vi "Calculate_WDID.vi"() -> ()   [LabVIEW 2012]
panel:
  in  "SID":u32=9
  in  "ST":u32=12
  in  "DT":u32
  in  "DU":u32=17
  in  "CV":u32
  out "WDID (binair)":u32 format="%032b"
  out "WDID (decimal)":u32
  # "This VI calculates WDID-word (32 bits unsigned integer)."
  # "// Creates a Weather Data ID from the components\n#define MAKE_WDID(CV, DU, DT, ST, SID)  ( ((CV) & 0x1F) | (((DU) & 0x1F)<<5) | (((DT) & 0x1F)<<10) | (((ST) & 0xFF)<<16) | (((SID) & 0xFF) <<24) )\n\n// Weather Data ID field values\n\n// Calculated Variable - 5 bits        // Input parameters\n#define WDAT_CV_DIRECT_DATA      (0)   // NOT a calculated value, \n                                       // 0=SID   1=ST\n#define WDAT_CV_DEWPOINT         (1)   // 0-Temp, 1-Humidity\n#define WDAT_CV_WINDCHILL        (2)   // 0-Temp,             Implied: Wind Speed\n#define WDAT_CV_HEAT             (3)   // 0-Temp, 1-Humidity\n#define WDAT_CV_THWINDEX         (4)   // 0-Temp, 1-Humidity, Implied: Wind Speed\n#define WDAT_CV_THSWINDEX        (5)   // 0-Temp, 1-Humidity, Implied: Speed, Solar, Time/Location\n#define WDAT_CV_WETBULB          (6)   // 0-Temp, 1-Humidity\n#define WDAT_CV_WINDRUN          (7)   //                     Implied: Speed, Arc Interval\n#define WDAT_CV_DEGDAYS_INTEG    (8)   // 0-Temp, 1-Threshold Implied: Arc Interval\n#define WDAT_CV_SOLAR_ENERGY     (9)   //                     Implied: Solar, Arc Interval\n#define WDAT_CV_UV_DOSE          (10)  //                     Implied: UV, Arc Interval\n#define WDAT_CV_AIR_DENSITY      (11)  // 0-Temp, 1-Humidity  Implied barometer\n#define WDAT_CV_EMC              (12)  // 0-Temp, 1-Humidity\n#define WDAT_CV_ET               (13)  // This is calculated on the Vantage, but does not have \n                                       // a particular sensor to file it under\n#define WDAT_CV_DEGDAYS_HI_LOW   (14)  // 0-Temp, 1-Threshold Implied: Arc Interval\n\n// Display Units - 5 bits - This is NOT an independant variable\n#define WDAT_DU_TEMP_DEG         (0)   // Degrees of Temperature (F,C)\n#define WDAT_DU_DEG_DAYS         (1)   // Degrees of Temp Accumulation (0F = 0C)\n#define WD0      (2)   // Water Accumulation (Rain, ET) (in,mm)\n#define WDAT_DU_WATER_ACCUM      (2)   // Water Accumulation (Rain, ET) (in,mm) -- another define\n#define WDAT_DU_WATER_RATE       (3)   // Water Rate (in/hr, mm/hr)\n#define WDAT_DU_SPEED            (4)   // Wind Speed (mph,kt,kph,m/s)\n#define WDAT_DU_DIR_DEG          (5)   // Wind Direction in degrees \n#define WDAT_DU_DIR_SECTOR       (6)   // Wind Direction in sector code\n#define WDAT_DU_PRESSURE         (7)   // Air Pressure (in Hg, mm Hg, mb)\n#define WDAT_DU_TIME             (8)   // Time of Day (12hr, 24hr)\n#define WDAT_DU_TIME_ACCUM       (9)   // Accumulated # minutes\n#define WDAT_DU_SOLAR_RAD        (10)  // Solar Rad (W/m^2)\n#define WDAT_DU_SOLAR_ENERGY     (11)  // Solar Energy (Ly)\n#define WDAT_DU_UV_INDEX         (12)  // UV radiation (Index)\n#define WDAT_DU_UV_DOSE          (13)  // UV Dose (MEDs)\n#define WDAT_DU_PERCENT          (14)  // Percentage (i.e. Relative Hum) (%)\n#define WDAT_DU_SOIL_MOISTURE    (15)  // Wetness of the Soil (cb)\n#define WDAT_DU_LEAF_WET         (16)  // Wetness of Leaf surface (0-15)\n#define WDAT_DU_SCALAR           (17)  // Dimensionless numbers (Reed Open, nSamples, etc)\n#define WDAT_DU_DISTANCE         (18)  // Miles, Km, etc for Wind run\n#define WDAT_DU_ELEVATION        (19)  // Feet or Meters. for Bar Calibration etc\n#define WDAT_DU_AIR_DENSITY      (20)  // Air density units\n#define WDAT_DU_BAR_TREND        (21)  // barometer trend (5-position)\n\n// Data Type - 5 bits\n#define WDAT_DT_CURRENT          (0)   // Current instantanious value\n//#define WDAT_DT_ARC_ACCUM        (1)   // Accumulation over the archive interval\n//#define WDAT_DT_HIGH             (2)   // High within an archive interval\n//#define WDAT_DT_LOW              (3)   // Low within an archive interval\n#define WDAT_DT_DAY_HIGH         (4)   // Daily High\n//#define WDAT_DT_DAY_HIGH_TIME    (5)   // Time of Daily High\n#define WDAT_DT_DAY_LOW          (6)   // Daily Low\n//#define WDAT_DT_DAY_LOW_TIME     (7)   // Time of Daily Low\n#define WDAT_DT_DAY_AVERAGE      (8)   // Daily Average\n#define WDAT_DT_DAY_ACCUM        (9)   // Daily Accumulation\n#define WDAT_DT_MONTH_HIGH       (10)  // Monthly High\n//#define WDAT_DT_MONTH_HIGH_TIME  (11)  // Time of Monthly High\n#define WDAT_DT_MONTH_LOW        (12)  // Monthly Low\n//#define WDAT_DT_MONTH_LOW_TIME   (13)  // Time of Monthly Low\n//#define WDAT_DT_MONTH_AVERAGE    (14)  // Monthly Average\n//#define WDAT_DT_MONTH_AVG_HIGH   (15)  // Monthly Average of Daily Highs\n//#define WDAT_DT_MONTH_AVG_LOW    (16)  // Monthly Average of Daily Lows\n//#define WDAT_DT_MONTH_HIGH_AVG   (17)  // Monthly High of Daily Averages\n//#define WDAT_DT_MONTH_LOW_AVG    (18)  // Monthly Low of Daily Averages\n#define WDAT_DT_YEAR_HIGH        (19)  // Yearly high value\n#define WDAT_DT_YEAR_LOW         (20)  // Yearly low value\n#define WDAT_DT_STORM_ACCUM      (21)  // Month Accumulation\n#define WDAT_DT_MONTH_ACCUM      (22)  // Month Accumulation\n#define WDAT_DT_YEAR_ACCUM       (23)  // Year Accumulation\n#define WDAT_DT_HOUR_HIGH        (24)  // Hourly High (Rain Rate Only)\n// New for Loop 2\n#define WDAT_DT_2MIN_AVG              (25)    // 2 Min Wind speed \n#define WDAT_DT_10MIN_HIGH            (26)    // 10 Min Wind gust\n#define WDAT_DT_1HR_ACCUM             (27)    // Last hour rain\n#define WDAT_DT_24HR_ACCUM            (28)    // Last 24 hour rain\n\n\n// Sensor Type -- or Parameter 1 in calculated values - 8 bits\n#define WDAT_ST_TEMPERATURE      (0)\n#define WDAT_ST_HUMIDITY         (1)\n#define WDAT_ST_SPEED            (2)\n#define WDAT_ST_DIRECTION        (3)\n#define WDAT_ST_BAROMETER        (4)\n#define WDAT_ST_RAIN             (5)\n#define WDAT_ST_RAIN_RATE        (6)\n#define WDAT_ST_SOLAR            (7)\n#define WDAT_ST_UV               (8)\n#define WDAT_ST_SOIL             (9)\n#define WDAT_ST_LEAF             (10)\n#define WDAT_ST_TIME             (11)\n#define WDAT_ST_NUMBER           (12)  // various dimensionless numbers\n\n\n// Sensor ID (Temperature, Humidity, Soil, Leaf, Wind Speed?) - 8 bits\n//  The meaning of these values depends on the Sensor Type\n// Temp and Hum  values\n#define WDAT_SID_TH_OUTSIDE      (0)\n#define WDAT_SID_TH_INSIDE       (1)\n#define WDAT_SID_TH_EX_2         (2)\n#define WDAT_SID_TH_EX_3         (3)\n#define WDAT_SID_TH_EX_4         (4)\n#define WDAT_SID_TH_EX_5         (5)\n#define WDAT_SID_TH_EX_6         (6)\n#define WDAT_SID_TH_EX_7         (7)\n#define WDAT_SID_TH_EX_8         (8)\n\n// Temp, Soil (use the same id for temp and moisture)\n#define WDAT_SID_T_SOIL_1        (9)\n#define WDAT_SID_T_SOIL_2        (10)\n#define WDAT_SID_T_SOIL_3        (11)\n#define WDAT_SID_T_SOIL_4        (12)\n//#define WDAT_SID_T_SOIL_5        (13)  // not used in DLL\n//#define WDAT_SID_T_SOIL_6        (14)  // not used in DLL\n\n// leaf wetness\n#define WDAT_SID_T_LEAF_1        (15)\n#define WDAT_SID_T_LEAF_2        (16)\n//#define WDAT_SID_T_LEAF_3        (17)  // not used in DLL\n//#define WDAT_SID_T_LEAF_4        (18)  // not used in DLL\n\n// Wind Speed\n#define WDAT_SID_WIND_SPEED      (0)\n#define WDAT_SID_WIND_10_MIN     (1)\n\n// Barometer\n#define WDAT_SID_BAR_SEA_LEVEL   (0)\n#define WDAT_SID_BAR_STATION     (1)\n#define WDAT_SID_BAR_ALTIMETER   (2)    // Vue Altimeter\n\n// Scalar Values use these IDs\n//#define WDAT_SID_ARC_PERIOD      (0)  // not used in DLL\n//#define WDAT_SID_TX_ID           (1)  // not used in DLL\n//#define WDAT_SID_WIND_SAMPLES    (2)  // not used in DLL\n//#define WDAT_SID_RECEPTION       (3)  // not used in DLL\n//#define WDAT_SID_REED_OPEN       (4)  // not used in DLL\n//#define WDAT_SID_REED_CLOSED     (5)  // not used in DLL\n//#define WDAT_SID_REED_CYCLE      (6)  // not used in DLL\n#define WDAT_SID_REC_TIME        (7)\n//#define WDAT_SID_EXP_WIND_SAMPLES (8)  // not used in DLL\n#define WDAT_SID_CON_BATT        (9)\n#define WDAT_SID_TX_BATT         (10)\n#define WDAT_SID_REP_BATT        (11)\n#define WDAT_SID_FORECAST_CODE   (12)\n#define WDAT_SID_FORECAST_ICON   (13)\n\n// accumulated time values\n#define WDAT_SID_DATA_SPAN       (0)  // not used in DLL\n#define WDAT_SID_MIN_SUN         (1)  // not used in DLL\n#define WDAT_SID_SUNRISE         (2)\n#define WDAT_SID_SUNSET          (3)\n\n//#define WDAT_SID_\n//#define WDAT_SID_\n\n// Anything Else\n#define WDAT_SID_DEFAULT_SENSOR        (0)\n#define WDAT_SID_EXTRA_RAD_SENSOR      (1)   // used for THSW Index calculation\n\n\n// predefined sensor values\n\n// outside temperature\n#define CUR_OUT_TEMP_WDID        MAKE_WDID(WDAT_CV_DIRECT_DATA, WDAT_DU_TEMP_DEG, WDAT_DT_CURRENT,   WDAT_ST_TEMPERATURE, WDAT_SID_TH_OUTSIDE)    \n#define DAY_HI_OUT_TEMP_WDID     MAKE_WDID(WDAT_CV_DIRECT_DATA, WDAT_DU_TEMP_DEG, WDAT_DT_DAY_HIGH,  WDAT_ST_TEMPERATURE, WDAT_SID_TH_OUTSIDE)    \n#define DAY_LOW_OUT_TEMP_WDID    MAKE_WDID(WDAT_CV_DIRECT_DATA, WDAT_DU_TEMP_DEG, WDAT_DT_DAY_LOW,   WDAT_ST_TEMPERATURE, WDAT_SID_TH_OUTSIDE)    \n#define MONTH_HI_OUT_TEMP_WDID   MAKE_WDID(WDAT_CV_DIRECT_DATA, WDAT_DU_TEMP_DEG, WDAT_DT_MONTH_HIGH,WDAT_ST_TEMPERATURE, WDAT_SID_TH_OUTSIDE)    \n#define MONTH_LOW_OUT_TEMP_WDID  MAKE_WDID(WDAT_CV_DIRECT_DATA, WDAT_DU_TEMP_DEG, WDAT_DT_MONTH_LOW, WDAT_ST_TEMPERATURE, WDAT_SID_TH_OUTSIDE)    \n#define YEAR_HI_OUT_TEMP_WDID    MAKE_WDID(WDAT_CV_DIRECT_DATA, WDAT_DU_TEMP_DEG, WDAT_DT_YEAR_HIGH, WDAT_ST_TEMPERATURE, WDAT_SID_TH_OUTSIDE)    \n#define YEAR_LOW_OUT_TEMP_WDID   MAKE_WDID(WDAT_CV_DIRECT_DATA, WDAT_DU_TEMP_DEG, WDAT_DT_YEAR_LOW,  WDAT_ST_TEMPERATURE, WDAT_SID_TH_OUTSIDE)    \n\n// inside temperature\n#define CUR_IN_TEMP_WDID         MAKE_WDID(WDAT_CV_DIRECT_DATA, WDAT_DU_TEMP_DEG, WDAT_DT_CURRENT,   WDAT_ST_TEMPERATURE, WDAT_SID_TH_INSIDE)    \n#define DAY_HI_IN_TEMP_WDID      MAKE_WDID(WDAT_CV_DIRECT_DATA, WDAT_DU_TEMP_DEG, WDAT_DT_DAY_HIGH,  WDAT_ST_TEMPERATURE, WDAT_SID_TH_INSIDE)    \n#define DAY_LOW_IN_TEMP_WDID     MAKE_WDID(WDAT_CV_DIRECT_DATA, WDAT_DU_TEMP_DEG, WDAT_DT_DAY_LOW,   WDAT_ST_TEMPERATURE, WDAT_SID_TH_INSIDE)    \n#define MONTH_HI_IN_TEMP_WDID    MAKE_WDID(WDAT_CV_DIRECT_DATA, WDAT_DU_TEMP_DEG, WDAT_DT_MONTH_HIGH,WDAT_ST_TEMPERATURE, WDAT_SID_TH_INSIDE)    \n#define MONTH_LOW_IN_TEMP_WDID   MAKE_WDID(WDAT_CV_DIRECT_DATA, WDAT_DU_TEMP_DEG, WDAT_DT_MONTH_LOW, WDAT_ST_TEMPERATURE, WDAT_SID_TH_INSIDE)    \n#define YEAR_HI_IN_TEMP_WDID     MAKE_WDID(WDAT_CV_DIRECT_DATA, WDAT_DU_TEMP_DEG, WDAT_DT_YEAR_HIGH, WDAT_ST_TEMPERATURE, WDAT_SID_TH_INSIDE)    \n#define YEAR_LOW_IN_TEMP_WDID    MAKE_WDID(WDAT_CV_DIRECT_DATA, WDAT_DU_TEMP_DEG, WDAT_DT_YEAR_LOW,  WDAT_ST_TEMPERATURE, WDAT_SID_TH_INSIDE)    \n\n// Out humidity\n#define CUR_OUT_HUM_WDID         MAKE_WDID(WDAT_CV_DIRECT_DATA, WDAT_DU_PERCENT,  WDAT_DT_CURRENT,   WDAT_ST_HUMIDITY,    WDAT_SID_TH_OUTSIDE)    \n#define DAY_HI_OUT_HUM_WDID      MAKE_WDID(WDAT_CV_DIRECT_DATA, WDAT_DU_PERCENT,  WDAT_DT_DAY_HIGH,  WDAT_ST_HUMIDITY,    WDAT_SID_TH_OUTSIDE)    \n#define DAY_LOW_OUT_HUM_WDID     MAKE_WDID(WDAT_CV_DIRECT_DATA, WDAT_DU_PERCENT,  WDAT_DT_DAY_LOW,   WDAT_ST_HUMIDITY,    WDAT_SID_TH_OUTSIDE)    \n#define MONTH_HI_OUT_HUM_WDID    MAKE_WDID(WDAT_CV_DIRECT_DATA, WDAT_DU_PERCENT,  WDAT_DT_MONTH_HIGH,WDAT_ST_HUMIDITY,    WDAT_SID_TH_OUTSIDE)    \n#define MONTH_LOW_OUT_HUM_WDID   MAKE_WDID(WDAT_CV_DIRECT_DATA, WDAT_DU_PERCENT,  WDAT_DT_MONTH_LOW, WDAT_ST_HUMIDITY,    WDAT_SID_TH_OUTSIDE)    \n#define YEAR_HI_OUT_HUM_WDID     MAKE_WDID(WDAT_CV_DIRECT_DATA, WDAT_DU_PERCENT,  WDAT_DT_YEAR_HIGH, WDAT_ST_HUMIDITY,    WDAT_SID_TH_OUTSIDE)    \n#define YEAR_LOW_OUT_HUM_WDID    MAKE_WDID(WDAT_CV_DIRECT_DATA, WDAT_DU_PERCENT,  WDAT_DT_YEAR_LOW,  WDAT_ST_HUMIDITY,    WDAT_SID_TH_OUTSIDE)    \n\n// In humidity\n#define CUR_IN_HUM_WDID          MAKE_WDID(WDAT_CV_DIRECT_DATA, WDAT_DU_PERCENT,  WDAT_DT_CURRENT,   WDAT_ST_HUMIDITY,    WDAT_SID_TH_INSIDE)    \n#define DAY_HI_IN_HUM_WDID       MAKE_WDID(WDAT_CV_DIRECT_DATA, WDAT_DU_PERCENT,  WDAT_DT_DAY_HIGH,  WDAT_ST_HUMIDITY,    WDAT_SID_TH_INSIDE)    \n#define DAY_LOW_IN_HUM_WDID      MAKE_WDID(WDAT_CV_DIRECT_DATA, WDAT_DU_PERCENT,  WDAT_DT_DAY_LOW,   WDAT_ST_HUMIDITY,    WDAT_SID_TH_INSIDE)    \n#define MONTH_HI_IN_HUM_WDID     MAKE_WDID(WDAT_CV_DIRECT_DATA, WDAT_DU_PERCENT,  WDAT_DT_MONTH_HIGH,WDAT_ST_HUMIDITY,    WDAT_SID_TH_INSIDE)    \n#define MONTH_LOW_IN_HUM_WDID    MAKE_WDID(WDAT_CV_DIRECT_DATA, WDAT_DU_PERCENT,  WDAT_DT_MONTH_LOW, WDAT_ST_HUMIDITY,    WDAT_SID_TH_INSIDE)    \n#define YEAR_HI_IN_HUM_WDID      MAKE_WDID(WDAT_CV_DIRECT_DATA, WDAT_DU_PERCENT,  WDAT_DT_YEAR_HIGH, WDAT_ST_HUMIDITY,    WDAT_SID_TH_INSIDE)    \n#define YEAR_LOW_IN_HUM_WDID     MAKE_WDID(WDAT_CV_DIRECT_DATA, WDAT_DU_PERCENT,  WDAT_DT_YEAR_LOW,  WDAT_ST_HUMIDITY,    WDAT_SID_TH_INSIDE)    \n\n// Dew point\n#define CUR_OUT_DEW_WDID         MAKE_WDID(WDAT_CV_DEWPOINT,    WDAT_DU_TEMP_DEG, WDAT_DT_CURRENT,   WDAT_SID_TH_OUTSIDE, WDAT_SID_TH_OUTSIDE)\n#define DAY_HI_OUT_DEW_WDID      MAKE_WDID(WDAT_CV_DEWPOINT,    WDAT_DU_TEMP_DEG, WDAT_DT_DAY_HIGH,  WDAT_SID_TH_OUTSIDE, WDAT_SID_TH_OUTSIDE)\n#define DAY_LOW_OUT_DEW_WDID     MAKE_WDID(WDAT_CV_DEWPOINT,    WDAT_DU_TEMP_DEG, WDAT_DT_DAY_LOW,   WDAT_SID_TH_OUTSIDE, WDAT_SID_TH_OUTSIDE)\n#define MONTH_HI_OUT_DEW_WDID    MAKE_WDID(WDAT_CV_DEWPOINT,    WDAT_DU_TEMP_DEG, WDAT_DT_MONTH_HIGH,WDAT_SID_TH_OUTSIDE, WDAT_SID_TH_OUTSIDE)\n#define MONTH_LOW_OUT_DEW_WDID   MAKE_WDID(WDAT_CV_DEWPOINT,    WDAT_DU_TEMP_DEG, WDAT_DT_MONTH_LOW, WDAT_SID_TH_OUTSIDE, WDAT_SID_TH_OUTSIDE)\n#define YEAR_HI_OUT_DEW_WDID     MAKE_WDID(WDAT_CV_DEWPOINT,    WDAT_DU_TEMP_DEG, WDAT_DT_YEAR_HIGH, WDAT_SID_TH_OUTSIDE, WDAT_SID_TH_OUTSIDE)\n#define YEAR_LOW_OUT_DEW_WDID    MAKE_WDID(WDAT_CV_DEWPOINT,    WDAT_DU_TEMP_DEG, WDAT_DT_YEAR_LOW,  WDAT_SID_TH_OUTSIDE, WDAT_SID_TH_OUTSIDE)\n\n// Wind Chill\n#define CUR_WIND_CHILL_WDID      MAKE_WDID(WDAT_CV_WINDCHILL,   WDAT_DU_TEMP_DEG, WDAT_DT_CURRENT,   0,                   WDAT_SID_TH_OUTSIDE)    \n#define DAY_LOW_WIND_CHILL_WDID  MAKE_WDID(WDAT_CV_WINDCHILL,   WDAT_DU_TEMP_DEG, WDAT_DT_DAY_LOW,   0,                   WDAT_SID_TH_OUTSIDE)    \n#define MONTH_LOW_WIND_CHILL_WDID MAKE_WDID(WDAT_CV_WINDCHILL,  WDAT_DU_TEMP_DEG, WDAT_DT_MONTH_LOW, 0,                   WDAT_SID_TH_OUTSIDE)    \n#define YEAR_LOW_WIND_CHILL_WDID MAKE_WDID(WDAT_CV_WINDCHILL,   WDAT_DU_TEMP_DEG, WDAT_DT_YEAR_LOW,  0,                   WDAT_SID_TH_OUTSIDE)    \n\n// Heat Index\n#define CUR_OUT_HEAT_WDID        MAKE_WDID(WDAT_CV_HEAT,        WDAT_DU_TEMP_DEG, WDAT_DT_CURRENT,   WDAT_SID_TH_OUTSIDE, WDAT_SID_TH_OUTSIDE)    \n#define DAY_HI_OUT_HEAT_WDID     MAKE_WDID(WDAT_CV_HEAT,        WDAT_DU_TEMP_DEG, WDAT_DT_DAY_HIGH,  WDAT_SID_TH_OUTSIDE, WDAT_SID_TH_OUTSIDE)    \n#define MONTH_HI_OUT_HEAT_WDID   MAKE_WDID(WDAT_CV_HEAT,        WDAT_DU_TEMP_DEG, WDAT_DT_MONTH_HIGH,WDAT_SID_TH_OUTSIDE, WDAT_SID_TH_OUTSIDE)    \n#define YEAR_HI_OUT_HEAT_WDID    MAKE_WDID(WDAT_CV_HEAT,        WDAT_DU_TEMP_DEG, WDAT_DT_YEAR_HIGH, WDAT_SID_TH_OUTSIDE, WDAT_SID_TH_OUTSIDE)    \n\n// THW Index - current data only\n#define CUR_THW_INDEX_WDID       MAKE_WDID(WDAT_CV_THWINDEX,    WDAT_DU_TEMP_DEG, WDAT_DT_CURRENT,   WDAT_SID_TH_OUTSIDE, WDAT_SID_TH_OUTSIDE)    \n\n// THSW Index\n#define CUR_THSW_INDEX_WDID      MAKE_WDID(WDAT_CV_THSWINDEX,   WDAT_DU_TEMP_DEG, WDAT_DT_CURRENT,   WDAT_SID_TH_OUTSIDE, WDAT_SID_TH_OUTSIDE)    \n#define DAY_HI_THSW_INDEX_WDID   MAKE_WDID(WDAT_CV_THSWINDEX,   WDAT_DU_TEMP_DEG, WDAT_DT_DAY_HIGH,  WDAT_SID_TH_OUTSIDE, WDAT_SID_TH_OUTSIDE)    \n#define MONTH_HI_THSW_INDEX_WDID MAKE_WDID(WDAT_CV_THSWINDEX, WDAT_DU_TEMP_DEG, WDAT_DT_MONTH_HIGH,WDAT_SID_TH_OUTSIDE, WDAT_SID_TH_OUTSIDE)    \n#define YEAR_HI_THSW_INDEX_WDID  MAKE_WDID(WDAT_CV_THSWINDEX,  WDAT_DU_TEMP_DEG, WDAT_DT_YEAR_HIGH, WDAT_SID_TH_OUTSIDE, WDAT_SID_TH_OUTSIDE)    \n\n// inside Dew and Heat values - current data only\n#define CUR_IN_DEW_WDID          MAKE_WDID(WDAT_CV_DEWPOINT,    WDAT_DU_TEMP_DEG, WDAT_DT_CURRENT,   WDAT_SID_TH_INSIDE,  WDAT_SID_TH_INSIDE)    \n#define CUR_IN_HEAT_WDID         MAKE_WDID(WDAT_CV_HEAT,        WDAT_DU_TEMP_DEG, WDAT_DT_CURRENT,   WDAT_SID_TH_INSIDE,  WDAT_SID_TH_INSIDE)\n\n// instantanious Wind Speed\n#define CUR_SPEED_WDID           MAKE_WDID(WDAT_CV_DIRECT_DATA, WDAT_DU_SPEED,    WDAT_DT_CURRENT,   WDAT_ST_SPEED,     WDAT_SID_WIND_SPEED)    \n#define DAY_HI_SPEED_WDID        MAKE_WDID(WDAT_CV_DIRECT_DATA, WDAT_DU_SPEED,    WDAT_DT_DAY_HIGH,  WDAT_ST_SPEED,     WDAT_SID_WIND_SPEED)    \n#define MONTH_HI_SPEED_WDID      MAKE_WDID(WDAT_CV_DIRECT_DATA, WDAT_DU_SPEED,    WDAT_DT_MONTH_HIGH,WDAT_ST_SPEED,     WDAT_SID_WIND_SPEED)    \n#define YEAR_HI_SPEED_WDID       MAKE_WDID(WDAT_CV_DIRECT_DATA, WDAT_DU_SPEED,    WDAT_DT_YEAR_HIGH, WDAT_ST_SPEED,     WDAT_SID_WIND_SPEED)    \n\n// wind values\n#define CUR_AVG_SPEED_WDID       MAKE_WDID(WDAT_CV_DIRECT_DATA, WDAT_DU_SPEED,    WDAT_DT_CURRENT,   WDAT_ST_SPEED,     WDAT_SID_WIND_10_MIN)    \n\n//wind Direction\n#define CUR_WIND_DIR_WDID        MAKE_WDID(WDAT_CV_DIRECT_DATA, WDAT_DU_DIR_DEG,  WDAT_DT_CURRENT,   WDAT_ST_DIRECTION, WDAT_SID_WIND_SPEED)    \n#define CUR_WIND_DIR_SECTOR_WDID MAKE_WDID(WDAT_CV_DIRECT_DATA, WDAT_DU_DIR_SECTOR, WDAT_DT_CURRENT, WDAT_ST_DIRECTION, WDAT_SID_WIND_SPEED)    \n//#define CUR_DIR_OF_GUST_WDID     MAKE_WDID(WDAT_CV_DIRECT_DATA, WDAT_DU_DIR_SECTOR, WDAT_DT_HIGH,    WDAT_ST_DIRECTION, WDAT_SID_WIND_SPEED)    \n\n//#define CUR_WIND_RUN_WDID        MAKE_WDID(WDAT_CV_WINDRUN,     WDAT_DU_DISTANCE,   WDAT_DT_ARC_ACCUM, WDAT_ST_SPEED,   WDAT_SID_WIND_SPEED)    \n\n// barometer values\n#define CUR_SEA_LEV_BAR_WDID     MAKE_WDID(WDAT_CV_DIRECT_DATA, WDAT_DU_PRESSURE, WDAT_DT_CURRENT,   WDAT_ST_BAROMETER, WDAT_SID_BAR_SEA_LEVEL)    \n#define DAY_HI_SEA_LEV_BAR_WDID  MAKE_WDID(WDAT_CV_DIRECT_DATA, WDAT_DU_PRESSURE, WDAT_DT_DAY_HIGH,  WDAT_ST_BAROMETER, WDAT_SID_BAR_SEA_LEVEL)    \n#define DAY_LOW_SEA_LEV_BAR_WDID MAKE_WDID(WDAT_CV_DIRECT_DATA, WDAT_DU_PRESSURE, WDAT_DT_DAY_LOW,   WDAT_ST_BAROMETER, WDAT_SID_BAR_SEA_LEVEL)    \n#define MONTH_HI_SEA_LEV_BAR_WDID  MAKE_WDID(WDAT_CV_DIRECT_DATA,WDAT_DU_PRESSURE,WDAT_DT_MONTH_HIGH,WDAT_ST_BAROMETER, WDAT_SID_BAR_SEA_LEVEL)    \n#define MONTH_LOW_SEA_LEV_BAR_WDID MAKE_WDID(WDAT_CV_DIRECT_DATA,WDAT_DU_PRESSURE,WDAT_DT_MONTH_LOW, WDAT_ST_BAROMETER, WDAT_SID_BAR_SEA_LEVEL)    \n#define YEAR_HI_SEA_LEV_BAR_WDID   MAKE_WDID(WDAT_CV_DIRECT_DATA,WDAT_DU_PRESSURE,WDAT_DT_YEAR_HIGH, WDAT_ST_BAROMETER, WDAT_SID_BAR_SEA_LEVEL)    \n#define YEAR_LOW_SEA_LEV_BAR_WDID  MAKE_WDID(WDAT_CV_DIRECT_DATA,WDAT_DU_PRESSURE,WDAT_DT_YEAR_LOW,  WDAT_ST_BAROMETER, WDAT_SID_BAR_SEA_LEVEL)    \n\n#define CUR_STATIOM_BAR_WDID     MAKE_WDID(WDAT_CV_DIRECT_DATA, WDAT_DU_PRESSURE, WDAT_DT_CURRENT,   WDAT_ST_BAROMETER, WDAT_SID_BAR_STATION)    \n#define CUR_SEA_LEV_BAR_TREND_WDID MAKE_WDID(WDAT_CV_DIRECT_DATA,WDAT_DU_BAR_TREND,WDAT_DT_CURRENT,  WDAT_ST_BAROMETER, WDAT_SID_BAR_SEA_LEVEL)    \n\n// rain totals\n#define DAY_RAIN_WDID            MAKE_WDID(WDAT_CV_DIRECT_DATA, WDAT_DU_WATER_ACCUM, WDAT_DT_DAY_ACCUM,  WDAT_ST_RAIN,  WDAT_SID_DEFAULT_SENSOR)    \n#define STORM_RAIN_WDID          MAKE_WDID(WDAT_CV_DIRECT_DATA, WDAT_DU_WATER_ACCUM, WDAT_DT_STORM_ACCUM,WDAT_ST_RAIN,  WDAT_SID_DEFAULT_SENSOR)    \n#define MONTH_RAIN_WDID          MAKE_WDID(WDAT_CV_DIRECT_DATA, WDAT_DU_WATER_ACCUM, WDAT_DT_MONTH_ACCUM,WDAT_ST_RAIN,  WDAT_SID_DEFAULT_SENSOR)    \n#define YEAR_RAIN_WDID           MAKE_WDID(WDAT_CV_DIRECT_DATA, WDAT_DU_WATER_ACCUM, WDAT_DT_YEAR_ACCUM, WDAT_ST_RAIN,  WDAT_SID_DEFAULT_SENSOR)    \n\n// rain rate\n#define CUR_RAIN_RATE_WDID       MAKE_WDID(WDAT_CV_DIRECT_DATA, WDAT_DU_WATER_RATE,  WDAT_DT_CURRENT,    WDAT_ST_RAIN_RATE, WDAT_SID_DEFAULT_SENSOR)    \n#define HOUR_HI_RATE_WDID        MAKE_WDID(WDAT_CV_DIRECT_DATA, WDAT_DU_WATER_RATE,  WDAT_DT_HOUR_HIGH,  WDAT_ST_RAIN_RATE, WDAT_SID_DEFAULT_SENSOR)    \n#define DAY_HI_RATE_WDID         MAKE_WDID(WDAT_CV_DIRECT_DATA, WDAT_DU_WATER_RATE,  WDAT_DT_DAY_HIGH,   WDAT_ST_RAIN_RATE, WDAT_SID_DEFAULT_SENSOR)    \n#define MONTH_HI_RATE_WDID       MAKE_WDID(WDAT_CV_DIRECT_DATA, WDAT_DU_WATER_RATE,  WDAT_DT_MONTH_HIGH, WDAT_ST_RAIN_RATE, WDAT_SID_DEFAULT_SENSOR)    \n#define YEAR_HI_RATE_WDID        MAKE_WDID(WDAT_CV_DIRECT_DATA, WDAT_DU_WATER_RATE,  WDAT_DT_YEAR_HIGH,  WDAT_ST_RAIN_RATE, WDAT_SID_DEFAULT_SENSOR)    \n\n// ET\n#define DAY_ET_WDID              MAKE_WDID(WDAT_CV_ET,       WDAT_DU_WATER_ACCUM, WDAT_DT_DAY_ACCUM,  WDAT_SID_DEFAULT_SENSOR, WDAT_SID_DEFAULT_SENSOR)    \n#define MONTH_ET_WDID            MAKE_WDID(WDAT_CV_ET,       WDAT_DU_WATER_ACCUM, WDAT_DT_MONTH_ACCUM,WDAT_SID_DEFAULT_SENSOR, WDAT_SID_DEFAULT_SENSOR)    \n#define YEAR_ET_WDID             MAKE_WDID(WDAT_CV_ET,       WDAT_DU_WATER_ACCUM, WDAT_DT_YEAR_ACCUM, WDAT_SID_DEFAULT_SENSOR, WDAT_SID_DEFAULT_SENSOR)    \n\n\n// Solar / UV values\n#define CUR_SOLAR_RAD_WDID       MAKE_WDID(WDAT_CV_DIRECT_DATA, WDAT_DU_SOLAR_RAD, WDAT_DT_CURRENT,    WDAT_ST_SOLAR, WDAT_SID_DEFAULT_SENSOR)    \n#define DAY_HI_SOLAR_RAD_WDID    MAKE_WDID(WDAT_CV_DIRECT_DATA, WDAT_DU_SOLAR_RAD, WDAT_DT_DAY_HIGH,   WDAT_ST_SOLAR, WDAT_SID_DEFAULT_SENSOR)    \n#define MONTH_HI_SOLAR_RAD_WDID  MAKE_WDID(WDAT_CV_DIRECT_DATA, WDAT_DU_SOLAR_RAD, WDAT_DT_MONTH_HIGH, WDAT_ST_SOLAR, WDAT_SID_DEFAULT_SENSOR)    \n#define YEAR_HI_SOLAR_RAD_WDID   MAKE_WDID(WDAT_CV_DIRECT_DATA, WDAT_DU_SOLAR_RAD, WDAT_DT_YEAR_HIGH,  WDAT_ST_SOLAR, WDAT_SID_DEFAULT_SENSOR)    \n\n//#define CUR_SOLAR_ENERGY_WDID    MAKE_WDID(WDAT_CV_SOLAR_ENERGY, WDAT_DU_SOLAR_ENERGY, WDAT_DT_ARC_ACCUM, WDAT_ST_SOLAR, WDAT_SID_DEFAULT_SENSOR)    \n//#define CUR_EXTRA_SOLAR_RAD_WDID MAKE_WDID(WDAT_CV_DIRECT_DATA,  WDAT_DU_SOLAR_RAD,    WDAT_DT_CURRENT,   WDAT_ST_SOLAR, WDAT_SID_EXTRA_RAD_SENSOR)    \n \n#define CUR_UV_WDID              MAKE_WDID(WDAT_CV_DIRECT_DATA, WDAT_DU_UV_INDEX, WDAT_DT_CURRENT,   WDAT_ST_UV,     WDAT_SID_DEFAULT_SENSOR)    \n#define DAY_HI_UV_WDID           MAKE_WDID(WDAT_CV_DIRECT_DATA, WDAT_DU_UV_INDEX, WDAT_DT_DAY_HIGH,  WDAT_ST_UV,     WDAT_SID_DEFAULT_SENSOR)    \n#define MONTH_HI_UV_WDID         MAKE_WDID(WDAT_CV_DIRECT_DATA, WDAT_DU_UV_INDEX, WDAT_DT_MONTH_HIGH,WDAT_ST_UV,     WDAT_SID_DEFAULT_SENSOR)    \n#define YEAR_HI_UV_WDID          MAKE_WDID(WDAT_CV_DIRECT_DATA, WDAT_DU_UV_INDEX, WDAT_DT_YEAR_HIGH, WDAT_ST_UV,     WDAT_SID_DEFAULT_SENSOR)    \n\n//#define CUR_UV_DOSE_WDID         MAKE_WDID(WDAT_CV_UV_DOSE,      WDAT_DU_UV_DOSE,   WDAT_DT_ARC_ACCUM, WDAT_ST_UV, WDAT_SID_DEFAULT_SENSOR)    \n\n// Extra Temperatures \n#define CUR_TEMP_2_WDID          MAKE_WDID(WDAT_CV_DIRECT_DATA, WDAT_DU_TEMP_DEG, WDAT_DT_CURRENT,   WDAT_ST_TEMPERATURE, WDAT_SID_TH_EX_2)    \n#define DAY_HI_TEMP_2_WDID       MAKE_WDID(WDAT_CV_DIRECT_DATA, WDAT_DU_TEMP_DEG, WDAT_DT_DAY_HIGH,  WDAT_ST_TEMPERATURE, WDAT_SID_TH_EX_2)    \n#define DAY_LOW_TEMP_2_WDID      MAKE_WDID(WDAT_CV_DIRECT_DATA, WDAT_DU_TEMP_DEG, WDAT_DT_DAY_LOW,   WDAT_ST_TEMPERATURE, WDAT_SID_TH_EX_2)    \n#define MONTH_HI_TEMP_2_WDID     MAKE_WDID(WDAT_CV_DIRECT_DATA, WDAT_DU_TEMP_DEG, WDAT_DT_MONTH_HIGH,WDAT_ST_TEMPERATURE, WDAT_SID_TH_EX_2)    \n#define MONTH_LOW_TEMP_2_WDID    MAKE_WDID(WDAT_CV_DIRECT_DATA, WDAT_DU_TEMP_DEG, WDAT_DT_MONTH_LOW, WDAT_ST_TEMPERATURE, WDAT_SID_TH_EX_2)    \n#define YEAR_HI_TEMP_2_WDID      MAKE_WDID(WDAT_CV_DIRECT_DATA, WDAT_DU_TEMP_DEG, WDAT_DT_YEAR_HIGH, WDAT_ST_TEMPERATURE, WDAT_SID_TH_EX_2)    \n#define YEAR_LOW_TEMP_2_WDID     MAKE_WDID(WDAT_CV_DIRECT_DATA, WDAT_DU_TEMP_DEG, WDAT_DT_YEAR_LOW,  WDAT_ST_TEMPERATURE, WDAT_SID_TH_EX_2)    \n\n#define CUR_TEMP_3_WDID          MAKE_WDID(WDAT_CV_DIRECT_DATA, WDAT_DU_TEMP_DEG, WDAT_DT_CURRENT,   WDAT_ST_TEMPERATURE, WDAT_SID_TH_EX_3)    \n#define DAY_HI_TEMP_3_WDID       MAKE_WDID(WDAT_CV_DIRECT_DATA, WDAT_DU_TEMP_DEG, WDAT_DT_DAY_HIGH,  WDAT_ST_TEMPERATURE, WDAT_SID_TH_EX_3)    \n#define DAY_LOW_TEMP_3_WDID      MAKE_WDID(WDAT_CV_DIRECT_DATA, WDAT_DU_TEMP_DEG, WDAT_DT_DAY_LOW,   WDAT_ST_TEMPERATURE, WDAT_SID_TH_EX_3)    \n#define MONTH_HI_TEMP_3_WDID     MAKE_WDID(WDAT_CV_DIRECT_DATA, WDAT_DU_TEMP_DEG, WDAT_DT_MONTH_HIGH,WDAT_ST_TEMPERATURE, WDAT_SID_TH_EX_3)    \n#define MONTH_LOW_TEMP_3_WDID    MAKE_WDID(WDAT_CV_DIRECT_DATA, WDAT_DU_TEMP_DEG, WDAT_DT_MONTH_LOW, WDAT_ST_TEMPERATURE, WDAT_SID_TH_EX_3)    \n#define YEAR_HI_TEMP_3_WDID      MAKE_WDID(WDAT_CV_DIRECT_DATA, WDAT_DU_TEMP_DEG, WDAT_DT_YEAR_HIGH, WDAT_ST_TEMPERATURE, WDAT_SID_TH_EX_3)    \n#define YEAR_LOW_TEMP_3_WDID     MAKE_WDID(WDAT_CV_DIRECT_DATA, WDAT_DU_TEMP_DEG, WDAT_DT_YEAR_LOW,  WDAT_ST_TEMPERATURE, WDAT_SID_TH_EX_3)    \n\n#define CUR_TEMP_4_WDID          MAKE_WDID(WDAT_CV_DIRECT_DATA, WDAT_DU_TEMP_DEG, WDAT_DT_CURRENT,   WDAT_ST_TEMPERATURE, WDAT_SID_TH_EX_4)    \n#define DAY_HI_TEMP_4_WDID       MAKE_WDID(WDAT_CV_DIRECT_DATA, WDAT_DU_TEMP_DEG, WDAT_DT_DAY_HIGH,  WDAT_ST_TEMPERATURE, WDAT_SID_TH_EX_4)    \n#define DAY_LOW_TEMP_4_WDID      MAKE_WDID(WDAT_CV_DIRECT_DATA, WDAT_DU_TEMP_DEG, WDAT_DT_DAY_LOW,   WDAT_ST_TEMPERATURE, WDAT_SID_TH_EX_4)    \n#define MONTH_HI_TEMP_4_WDID     MAKE_WDID(WDAT_CV_DIRECT_DATA, WDAT_DU_TEMP_DEG, WDAT_DT_MONTH_HIGH,WDAT_ST_TEMPERATURE, WDAT_SID_TH_EX_4)    \n#define MONTH_LOW_TEMP_4_WDID    MAKE_WDID(WDAT_CV_DIRECT_DATA, WDAT_DU_TEMP_DEG, WDAT_DT_MONTH_LOW, WDAT_ST_TEMPERATURE, WDAT_SID_TH_EX_4)    \n#define YEAR_HI_TEMP_4_WDID      MAKE_WDID(WDAT_CV_DIRECT_DATA, WDAT_DU_TEMP_DEG, WDAT_DT_YEAR_HIGH, WDAT_ST_TEMPERATURE, WDAT_SID_TH_EX_4)    \n#define YEAR_LOW_TEMP_4_WDID     MAKE_WDID(WDAT_CV_DIRECT_DATA, WDAT_DU_TEMP_DEG, WDAT_DT_YEAR_LOW,  WDAT_ST_TEMPERATURE, WDAT_SID_TH_EX_4)    \n\n#define CUR_TEMP_5_WDID          MAKE_WDID(WDAT_CV_DIRECT_DATA, WDAT_DU_TEMP_DEG, WDAT_DT_CURRENT,   WDAT_ST_TEMPERATURE, WDAT_SID_TH_EX_5)    \n#define DAY_HI_TEMP_5_WDID       MAKE_WDID(WDAT_CV_DIRECT_DATA, WDAT_DU_TEMP_DEG, WDAT_DT_DAY_HIGH,  WDAT_ST_TEMPERATURE, WDAT_SID_TH_EX_5)    \n#define DAY_LOW_TEMP_5_WDID      MAKE_WDID(WDAT_CV_DIRECT_DATA, WDAT_DU_TEMP_DEG, WDAT_DT_DAY_LOW,   WDAT_ST_TEMPERATURE, WDAT_SID_TH_EX_5)    \n#define MONTH_HI_TEMP_5_WDID     MAKE_WDID(WDAT_CV_DIRECT_DATA, WDAT_DU_TEMP_DEG, WDAT_DT_MONTH_HIGH,WDAT_ST_TEMPERATURE, WDAT_SID_TH_EX_5)    \n#define MONTH_LOW_TEMP_5_WDID    MAKE_WDID(WDAT_CV_DIRECT_DATA, WDAT_DU_TEMP_DEG, WDAT_DT_MONTH_LOW, WDAT_ST_TEMPERATURE, WDAT_SID_TH_EX_5)    \n#define YEAR_HI_TEMP_5_WDID      MAKE_WDID(WDAT_CV_DIRECT_DATA, WDAT_DU_TEMP_DEG, WDAT_DT_YEAR_HIGH, WDAT_ST_TEMPERATURE, WDAT_SID_TH_EX_5)    \n#define YEAR_LOW_TEMP_5_WDID     MAKE_WDID(WDAT_CV_DIRECT_DATA, WDAT_DU_TEMP_DEG, WDAT_DT_YEAR_LOW,  WDAT_ST_TEMPERATURE, WDAT_SID_TH_EX_5)    \n\n#define CUR_TEMP_6_WDID          MAKE_WDID(WDAT_CV_DIRECT_DATA, WDAT_DU_TEMP_DEG, WDAT_DT_CURRENT,   WDAT_ST_TEMPERATURE, WDAT_SID_TH_EX_6)    \n#define DAY_HI_TEMP_6_WDID       MAKE_WDID(WDAT_CV_DIRECT_DATA, WDAT_DU_TEMP_DEG, WDAT_DT_DAY_HIGH,  WDAT_ST_TEMPERATURE, WDAT_SID_TH_EX_6)    \n#define DAY_LOW_TEMP_6_WDID      MAKE_WDID(WDAT_CV_DIRECT_DATA, WDAT_DU_TEMP_DEG, WDAT_DT_DAY_LOW,   WDAT_ST_TEMPERATURE, WDAT_SID_TH_EX_6)    \n#define MONTH_HI_TEMP_6_WDID     MAKE_WDID(WDAT_CV_DIRECT_DATA, WDAT_DU_TEMP_DEG, WDAT_DT_MONTH_HIGH,WDAT_ST_TEMPERATURE, WDAT_SID_TH_EX_6)    \n#define MONTH_LOW_TEMP_6_WDID    MAKE_WDID(WDAT_CV_DIRECT_DATA, WDAT_DU_TEMP_DEG, WDAT_DT_MONTH_LOW, WDAT_ST_TEMPERATURE, WDAT_SID_TH_EX_6)    \n#define YEAR_HI_TEMP_6_WDID      MAKE_WDID(WDAT_CV_DIRECT_DATA, WDAT_DU_TEMP_DEG, WDAT_DT_YEAR_HIGH, WDAT_ST_TEMPERATURE, WDAT_SID_TH_EX_6)    \n#define YEAR_LOW_TEMP_6_WDID     MAKE_WDID(WDAT_CV_DIRECT_DATA, WDAT_DU_TEMP_DEG, WDAT_DT_YEAR_LOW,  WDAT_ST_TEMPERATURE, WDAT_SID_TH_EX_6)    \n\n#define CUR_TEMP_7_WDID          MAKE_WDID(WDAT_CV_DIRECT_DATA, WDAT_DU_TEMP_DEG, WDAT_DT_CURRENT,   WDAT_ST_TEMPERATURE, WDAT_SID_TH_EX_7)    \n#define DAY_HI_TEMP_7_WDID       MAKE_WDID(WDAT_CV_DIRECT_DATA, WDAT_DU_TEMP_DEG, WDAT_DT_DAY_HIGH,  WDAT_ST_TEMPERATURE, WDAT_SID_TH_EX_7)    \n#define DAY_LOW_TEMP_7_WDID      MAKE_WDID(WDAT_CV_DIRECT_DATA, WDAT_DU_TEMP_DEG, WDAT_DT_DAY_LOW,   WDAT_ST_TEMPERATURE, WDAT_SID_TH_EX_7)    \n#define MONTH_HI_TEMP_7_WDID     MAKE_WDID(WDAT_CV_DIRECT_DATA, WDAT_DU_TEMP_DEG, WDAT_DT_MONTH_HIGH,WDAT_ST_TEMPERATURE, WDAT_SID_TH_EX_7)    \n#define MONTH_LOW_TEMP_7_WDID    MAKE_WDID(WDAT_CV_DIRECT_DATA, WDAT_DU_TEMP_DEG, WDAT_DT_MONTH_LOW, WDAT_ST_TEMPERATURE, WDAT_SID_TH_EX_7)    \n#define YEAR_HI_TEMP_7_WDID      MAKE_WDID(WDAT_CV_DIRECT_DATA, WDAT_DU_TEMP_DEG, WDAT_DT_YEAR_HIGH, WDAT_ST_TEMPERATURE, WDAT_SID_TH_EX_7)    \n#define YEAR_LOW_TEMP_7_WDID     MAKE_WDID(WDAT_CV_DIRECT_DATA, WDAT_DU_TEMP_DEG, WDAT_DT_YEAR_LOW,  WDAT_ST_TEMPERATURE, WDAT_SID_TH_EX_7)    \n\n#define CUR_TEMP_8_WDID          MAKE_WDID(WDAT_CV_DIRECT_DATA, WDAT_DU_TEMP_DEG, WDAT_DT_CURRENT,   WDAT_ST_TEMPERATURE, WDAT_SID_TH_EX_8)    \n#define DAY_HI_TEMP_8_WDID       MAKE_WDID(WDAT_CV_DIRECT_DATA, WDAT_DU_TEMP_DEG, WDAT_DT_DAY_HIGH,  WDAT_ST_TEMPERATURE, WDAT_SID_TH_EX_8)    \n#define DAY_LOW_TEMP_8_WDID      MAKE_WDID(WDAT_CV_DIRECT_DATA, WDAT_DU_TEMP_DEG, WDAT_DT_DAY_LOW,   WDAT_ST_TEMPERATURE, WDAT_SID_TH_EX_8)    \n#define MONTH_HI_TEMP_8_WDID     MAKE_WDID(WDAT_CV_DIRECT_DATA, WDAT_DU_TEMP_DEG, WDAT_DT_MONTH_HIGH,WDAT_ST_TEMPERATURE, WDAT_SID_TH_EX_8)    \n#define MONTH_LOW_TEMP_8_WDID    MAKE_WDID(WDAT_CV_DIRECT_DATA, WDAT_DU_TEMP_DEG, WDAT_DT_MONTH_LOW, WDAT_ST_TEMPERATURE, WDAT_SID_TH_EX_8)    \n#define YEAR_HI_TEMP_8_WDID      MAKE_WDID(WDAT_CV_DIRECT_DATA, WDAT_DU_TEMP_DEG, WDAT_DT_YEAR_HIGH, WDAT_ST_TEMPERATURE, WDAT_SID_TH_EX_8)    \n#define YEAR_LOW_TEMP_8_WDID     MAKE_WDID(WDAT_CV_DIRECT_DATA, WDAT_DU_TEMP_DEG, WDAT_DT_YEAR_LOW,  WDAT_ST_TEMPERATURE, WDAT_SID_TH_EX_8)    \n\n// Extra Humidities \n#define CUR_HUM_2_WDID           MAKE_WDID(WDAT_CV_DIRECT_DATA, WDAT_DU_PERCENT,  WDAT_DT_CURRENT,   WDAT_ST_HUMIDITY,    WDAT_SID_TH_EX_2)    \n#define DAY_HI_HUM_2_WDID        MAKE_WDID(WDAT_CV_DIRECT_DATA, WDAT_DU_PERCENT,  WDAT_DT_DAY_HIGH,  WDAT_ST_HUMIDITY,    WDAT_SID_TH_EX_2)    \n#define DAY_LOW_HUM_2_WDID       MAKE_WDID(WDAT_CV_DIRECT_DATA, WDAT_DU_PERCENT,  WDAT_DT_DAY_LOW,   WDAT_ST_HUMIDITY,    WDAT_SID_TH_EX_2)    \n#define MONTH_HI_HUM_2_WDID      MAKE_WDID(WDAT_CV_DIRECT_DATA, WDAT_DU_PERCENT,  WDAT_DT_MONTH_HIGH,WDAT_ST_HUMIDITY,    WDAT_SID_TH_EX_2)    \n#define MONTH_LOW_HUM_2_WDID     MAKE_WDID(WDAT_CV_DIRECT_DATA, WDAT_DU_PERCENT,  WDAT_DT_MONTH_LOW, WDAT_ST_HUMIDITY,    WDAT_SID_TH_EX_2)    \n#define YEAR_HI_HUM_2_WDID       MAKE_WDID(WDAT_CV_DIRECT_DATA, WDAT_DU_PERCENT,  WDAT_DT_YEAR_HIGH, WDAT_ST_HUMIDITY,    WDAT_SID_TH_EX_2)    \n#define YEAR_LOW_HUM_2_WDID      MAKE_WDID(WDAT_CV_DIRECT_DATA, WDAT_DU_PERCENT,  WDAT_DT_YEAR_LOW,  WDAT_ST_HUMIDITY,    WDAT_SID_TH_EX_2)    \n\n#define CUR_HUM_3_WDID           MAKE_WDID(WDAT_CV_DIRECT_DATA, WDAT_DU_PERCENT,  WDAT_DT_CURRENT,   WDAT_ST_HUMIDITY,    WDAT_SID_TH_EX_3)    \n#define DAY_HI_HUM_3_WDID        MAKE_WDID(WDAT_CV_DIRECT_DATA, WDAT_DU_PERCENT,  WDAT_DT_DAY_HIGH,  WDAT_ST_HUMIDITY,    WDAT_SID_TH_EX_3)    \n#define DAY_LOW_HUM_3_WDID       MAKE_WDID(WDAT_CV_DIRECT_DATA, WDAT_DU_PERCENT,  WDAT_DT_DAY_LOW,   WDAT_ST_HUMIDITY,    WDAT_SID_TH_EX_3)    \n#define MONTH_HI_HUM_3_WDID      MAKE_WDID(WDAT_CV_DIRECT_DATA, WDAT_DU_PERCENT,  WDAT_DT_MONTH_HIGH,WDAT_ST_HUMIDITY,    WDAT_SID_TH_EX_3)    \n#define MONTH_LOW_HUM_3_WDID     MAKE_WDID(WDAT_CV_DIRECT_DATA, WDAT_DU_PERCENT,  WDAT_DT_MONTH_LOW, WDAT_ST_HUMIDITY,    WDAT_SID_TH_EX_3)    \n#define YEAR_HI_HUM_3_WDID       MAKE_WDID(WDAT_CV_DIRECT_DATA, WDAT_DU_PERCENT,  WDAT_DT_YEAR_HIGH, WDAT_ST_HUMIDITY,    WDAT_SID_TH_EX_3)    \n#define YEAR_LOW_HUM_3_WDID      MAKE_WDID(WDAT_CV_DIRECT_DATA, WDAT_DU_PERCENT,  WDAT_DT_YEAR_LOW,  WDAT_ST_HUMIDITY,    WDAT_SID_TH_EX_3)    \n\n#define CUR_HUM_4_WDID           MAKE_WDID(WDAT_CV_DIRECT_DATA, WDAT_DU_PERCENT,  WDAT_DT_CURRENT,   WDAT_ST_HUMIDITY,    WDAT_SID_TH_EX_4)    \n#define DAY_HI_HUM_4_WDID        MAKE_WDID(WDAT_CV_DIRECT_DATA, WDAT_DU_PERCENT,  WDAT_DT_DAY_HIGH,  WDAT_ST_HUMIDITY,    WDAT_SID_TH_EX_4)    \n#define DAY_LOW_HUM_4_WDID       MAKE_WDID(WDAT_CV_DIRECT_DATA, WDAT_DU_PERCENT,  WDAT_DT_DAY_LOW,   WDAT_ST_HUMIDITY,    WDAT_SID_TH_EX_4)    \n#define MONTH_HI_HUM_4_WDID      MAKE_WDID(WDAT_CV_DIRECT_DATA, WDAT_DU_PERCENT,  WDAT_DT_MONTH_HIGH,WDAT_ST_HUMIDITY,    WDAT_SID_TH_EX_4)    \n#define MONTH_LOW_HUM_4_WDID     MAKE_WDID(WDAT_CV_DIRECT_DATA, WDAT_DU_PERCENT,  WDAT_DT_MONTH_LOW, WDAT_ST_HUMIDITY,    WDAT_SID_TH_EX_4)    \n#define YEAR_HI_HUM_4_WDID       MAKE_WDID(WDAT_CV_DIRECT_DATA, WDAT_DU_PERCENT,  WDAT_DT_YEAR_HIGH, WDAT_ST_HUMIDITY,    WDAT_SID_TH_EX_4)    \n#define YEAR_LOW_HUM_4_WDID      MAKE_WDID(WDAT_CV_DIRECT_DATA, WDAT_DU_PERCENT,  WDAT_DT_YEAR_LOW,  WDAT_ST_HUMIDITY,    WDAT_SID_TH_EX_4)    \n\n#define CUR_HUM_5_WDID           MAKE_WDID(WDAT_CV_DIRECT_DATA, WDAT_DU_PERCENT,  WDAT_DT_CURRENT,   WDAT_ST_HUMIDITY,    WDAT_SID_TH_EX_5)    \n#define DAY_HI_HUM_5_WDID        MAKE_WDID(WDAT_CV_DIRECT_DATA, WDAT_DU_PERCENT,  WDAT_DT_DAY_HIGH,  WDAT_ST_HUMIDITY,    WDAT_SID_TH_EX_5)    \n#define DAY_LOW_HUM_5_WDID       MAKE_WDID(WDAT_CV_DIRECT_DATA, WDAT_DU_PERCENT,  WDAT_DT_DAY_LOW,   WDAT_ST_HUMIDITY,    WDAT_SID_TH_EX_5)    \n#define MONTH_HI_HUM_5_WDID      MAKE_WDID(WDAT_CV_DIRECT_DATA, WDAT_DU_PERCENT,  WDAT_DT_MONTH_HIGH,WDAT_ST_HUMIDITY,    WDAT_SID_TH_EX_5)    \n#define MONTH_LOW_HUM_5_WDID     MAKE_WDID(WDAT_CV_DIRECT_DATA, WDAT_DU_PERCENT,  WDAT_DT_MONTH_LOW, WDAT_ST_HUMIDITY,    WDAT_SID_TH_EX_5)    \n#define YEAR_HI_HUM_5_WDID       MAKE_WDID(WDAT_CV_DIRECT_DATA, WDAT_DU_PERCENT,  WDAT_DT_YEAR_HIGH, WDAT_ST_HUMIDITY,    WDAT_SID_TH_EX_5)    \n#define YEAR_LOW_HUM_5_WDID      MAKE_WDID(WDAT_CV_DIRECT_DATA, WDAT_DU_PERCENT,  WDAT_DT_YEAR_LOW,  WDAT_ST_HUMIDITY,    WDAT_SID_TH_EX_5)    \n\n#define CUR_HUM_6_WDID           MAKE_WDID(WDAT_CV_DIRECT_DATA, WDAT_DU_PERCENT,  WDAT_DT_CURRENT,   WDAT_ST_HUMIDITY,    WDAT_SID_TH_EX_6)    \n#define DAY_HI_HUM_6_WDID        MAKE_WDID(WDAT_CV_DIRECT_DATA, WDAT_DU_PERCENT,  WDAT_DT_DAY_HIGH,  WDAT_ST_HUMIDITY,    WDAT_SID_TH_EX_6)    \n#define DAY_LOW_HUM_6_WDID       MAKE_WDID(WDAT_CV_DIRECT_DATA, WDAT_DU_PERCENT,  WDAT_DT_DAY_LOW,   WDAT_ST_HUMIDITY,    WDAT_SID_TH_EX_6)    \n#define MONTH_HI_HUM_6_WDID      MAKE_WDID(WDAT_CV_DIRECT_DATA, WDAT_DU_PERCENT,  WDAT_DT_MONTH_HIGH,WDAT_ST_HUMIDITY,    WDAT_SID_TH_EX_6)    \n#define MONTH_LOW_HUM_6_WDID     MAKE_WDID(WDAT_CV_DIRECT_DATA, WDAT_DU_PERCENT,  WDAT_DT_MONTH_LOW, WDAT_ST_HUMIDITY,    WDAT_SID_TH_EX_6)    \n#define YEAR_HI_HUM_6_WDID       MAKE_WDID(WDAT_CV_DIRECT_DATA, WDAT_DU_PERCENT,  WDAT_DT_YEAR_HIGH, WDAT_ST_HUMIDITY,    WDAT_SID_TH_EX_6)    \n#define YEAR_LOW_HUM_6_WDID      MAKE_WDID(WDAT_CV_DIRECT_DATA, WDAT_DU_PERCENT,  WDAT_DT_YEAR_LOW,  WDAT_ST_HUMIDITY,    WDAT_SID_TH_EX_6)    \n\n#define CUR_HUM_7_WDID           MAKE_WDID(WDAT_CV_DIRECT_DATA, WDAT_DU_PERCENT,  WDAT_DT_CURRENT,   WDAT_ST_HUMIDITY,    WDAT_SID_TH_EX_7)    \n#define DAY_HI_HUM_7_WDID        MAKE_WDID(WDAT_CV_DIRECT_DATA, WDAT_DU_PERCENT,  WDAT_DT_DAY_HIGH,  WDAT_ST_HUMIDITY,    WDAT_SID_TH_EX_7)    \n#define DAY_LOW_HUM_7_WDID       MAKE_WDID(WDAT_CV_DIRECT_DATA, WDAT_DU_PERCENT,  WDAT_DT_DAY_LOW,   WDAT_ST_HUMIDITY,    WDAT_SID_TH_EX_7)    \n#define MONTH_HI_HUM_7_WDID      MAKE_WDID(WDAT_CV_DIRECT_DATA, WDAT_DU_PERCENT,  WDAT_DT_MONTH_HIGH,WDAT_ST_HUMIDITY,    WDAT_SID_TH_EX_7)    \n#define MONTH_LOW_HUM_7_WDID     MAKE_WDID(WDAT_CV_DIRECT_DATA, WDAT_DU_PERCENT,  WDAT_DT_MONTH_LOW, WDAT_ST_HUMIDITY,    WDAT_SID_TH_EX_7)    \n#define YEAR_HI_HUM_7_WDID       MAKE_WDID(WDAT_CV_DIRECT_DATA, WDAT_DU_PERCENT,  WDAT_DT_YEAR_HIGH, WDAT_ST_HUMIDITY,    WDAT_SID_TH_EX_7)    \n#define YEAR_LOW_HUM_7_WDID      MAKE_WDID(WDAT_CV_DIRECT_DATA, WDAT_DU_PERCENT,  WDAT_DT_YEAR_LOW,  WDAT_ST_HUMIDITY,    WDAT_SID_TH_EX_7)    \n\n#define CUR_HUM_8_WDID           MAKE_WDID(WDAT_CV_DIRECT_DATA, WDAT_DU_PERCENT,  WDAT_DT_CURRENT,   WDAT_ST_HUMIDITY,    WDAT_SID_TH_EX_8)    \n#define DAY_HI_HUM_8_WDID        MAKE_WDID(WDAT_CV_DIRECT_DATA, WDAT_DU_PERCENT,  WDAT_DT_DAY_HIGH,  WDAT_ST_HUMIDITY,    WDAT_SID_TH_EX_8)    \n#define DAY_LOW_HUM_8_WDID       MAKE_WDID(WDAT_CV_DIRECT_DATA, WDAT_DU_PERCENT,  WDAT_DT_DAY_LOW,   WDAT_ST_HUMIDITY,    WDAT_SID_TH_EX_8)    \n#define MONTH_HI_HUM_8_WDID      MAKE_WDID(WDAT_CV_DIRECT_DATA, WDAT_DU_PERCENT,  WDAT_DT_MONTH_HIGH,WDAT_ST_HUMIDITY,    WDAT_SID_TH_EX_8)    \n#define MONTH_LOW_HUM_8_WDID     MAKE_WDID(WDAT_CV_DIRECT_DATA, WDAT_DU_PERCENT,  WDAT_DT_MONTH_LOW, WDAT_ST_HUMIDITY,    WDAT_SID_TH_EX_8)    \n#define YEAR_HI_HUM_8_WDID       MAKE_WDID(WDAT_CV_DIRECT_DATA, WDAT_DU_PERCENT,  WDAT_DT_YEAR_HIGH, WDAT_ST_HUMIDITY,    WDAT_SID_TH_EX_8)    \n#define YEAR_LOW_HUM_8_WDID      MAKE_WDID(WDAT_CV_DIRECT_DATA, WDAT_DU_PERCENT,  WDAT_DT_YEAR_LOW,  WDAT_ST_HUMIDITY,    WDAT_SID_TH_EX_8)    \n\n//Soil Moisture\n#define CUR_SOIL_M_1_WDID        MAKE_WDID(WDAT_CV_DIRECT_DATA, WDAT_DU_SOIL_MOISTURE, WDAT_DT_CURRENT,   WDAT_ST_SOIL,   WDAT_SID_T_SOIL_1)\n#define DAY_HI_SOIL_M_1_WDID     MAKE_WDID(WDAT_CV_DIRECT_DATA, WDAT_DU_SOIL_MOISTURE, WDAT_DT_DAY_HIGH,  WDAT_ST_SOIL,   WDAT_SID_T_SOIL_1)\n#define DAY_LOW_SOIL_M_1_WDID    MAKE_WDID(WDAT_CV_DIRECT_DATA, WDAT_DU_SOIL_MOISTURE, WDAT_DT_DAY_LOW,   WDAT_ST_SOIL,   WDAT_SID_T_SOIL_1)\n#define MONTH_HI_SOIL_M_1_WDID   MAKE_WDID(WDAT_CV_DIRECT_DATA, WDAT_DU_SOIL_MOISTURE, WDAT_DT_MONTH_HIGH,WDAT_ST_SOIL,   WDAT_SID_T_SOIL_1)\n#define MONTH_LOW_SOIL_M_1_WDID  MAKE_WDID(WDAT_CV_DIRECT_DATA, WDAT_DU_SOIL_MOISTURE, WDAT_DT_MONTH_LOW, WDAT_ST_SOIL,   WDAT_SID_T_SOIL_1)\n#define YEAR_HI_SOIL_M_1_WDID    MAKE_WDID(WDAT_CV_DIRECT_DATA, WDAT_DU_SOIL_MOISTURE, WDAT_DT_YEAR_HIGH, WDAT_ST_SOIL,   WDAT_SID_T_SOIL_1)\n#define YEAR_LOW_SOIL_M_1_WDID   MAKE_WDID(WDAT_CV_DIRECT_DATA, WDAT_DU_SOIL_MOISTURE, WDAT_DT_YEAR_LOW,  WDAT_ST_SOIL,   WDAT_SID_T_SOIL_1)\n\n#define CUR_SOIL_M_2_WDID        MAKE_WDID(WDAT_CV_DIRECT_DATA, WDAT_DU_SOIL_MOISTURE, WDAT_DT_CURRENT,   WDAT_ST_SOIL,   WDAT_SID_T_SOIL_2)\n#define DAY_HI_SOIL_M_2_WDID     MAKE_WDID(WDAT_CV_DIRECT_DATA, WDAT_DU_SOIL_MOISTURE, WDAT_DT_DAY_HIGH,  WDAT_ST_SOIL,   WDAT_SID_T_SOIL_2)\n#define DAY_LOW_SOIL_M_2_WDID    MAKE_WDID(WDAT_CV_DIRECT_DATA, WDAT_DU_SOIL_MOISTURE, WDAT_DT_DAY_LOW,   WDAT_ST_SOIL,   WDAT_SID_T_SOIL_2)\n#define MONTH_HI_SOIL_M_2_WDID   MAKE_WDID(WDAT_CV_DIRECT_DATA, WDAT_DU_SOIL_MOISTURE, WDAT_DT_MONTH_HIGH,WDAT_ST_SOIL,   WDAT_SID_T_SOIL_2)\n#define MONTH_LOW_SOIL_M_2_WDID  MAKE_WDID(WDAT_CV_DIRECT_DATA, WDAT_DU_SOIL_MOISTURE, WDAT_DT_MONTH_LOW, WDAT_ST_SOIL,   WDAT_SID_T_SOIL_2)\n#define YEAR_HI_SOIL_M_2_WDID    MAKE_WDID(WDAT_CV_DIRECT_DATA, WDAT_DU_SOIL_MOISTURE, WDAT_DT_YEAR_HIGH, WDAT_ST_SOIL,   WDAT_SID_T_SOIL_2)\n#define YEAR_LOW_SOIL_M_2_WDID   MAKE_WDID(WDAT_CV_DIRECT_DATA, WDAT_DU_SOIL_MOISTURE, WDAT_DT_YEAR_LOW,  WDAT_ST_SOIL,   WDAT_SID_T_SOIL_2)\n\n#define CUR_SOIL_M_3_WDID        MAKE_WDID(WDAT_CV_DIRECT_DATA, WDAT_DU_SOIL_MOISTURE, WDAT_DT_CURRENT,   WDAT_ST_SOIL,   WDAT_SID_T_SOIL_3)\n#define DAY_HI_SOIL_M_3_WDID     MAKE_WDID(WDAT_CV_DIRECT_DATA, WDAT_DU_SOIL_MOISTURE, WDAT_DT_DAY_HIGH,  WDAT_ST_SOIL,   WDAT_SID_T_SOIL_3)\n#define DAY_LOW_SOIL_M_3_WDID    MAKE_WDID(WDAT_CV_DIRECT_DATA, WDAT_DU_SOIL_MOISTURE, WDAT_DT_DAY_LOW,   WDAT_ST_SOIL,   WDAT_SID_T_SOIL_3)\n#define MONTH_HI_SOIL_M_3_WDID   MAKE_WDID(WDAT_CV_DIRECT_DATA, WDAT_DU_SOIL_MOISTURE, WDAT_DT_MONTH_HIGH,WDAT_ST_SOIL,   WDAT_SID_T_SOIL_3)\n#define MONTH_LOW_SOIL_M_3_WDID  MAKE_WDID(WDAT_CV_DIRECT_DATA, WDAT_DU_SOIL_MOISTURE, WDAT_DT_MONTH_LOW, WDAT_ST_SOIL,   WDAT_SID_T_SOIL_3)\n#define YEAR_HI_SOIL_M_3_WDID    MAKE_WDID(WDAT_CV_DIRECT_DATA, WDAT_DU_SOIL_MOISTURE, WDAT_DT_YEAR_HIGH, WDAT_ST_SOIL,   WDAT_SID_T_SOIL_3)\n#define YEAR_LOW_SOIL_M_3_WDID   MAKE_WDID(WDAT_CV_DIRECT_DATA, WDAT_DU_SOIL_MOISTURE, WDAT_DT_YEAR_LOW,  WDAT_ST_SOIL,   WDAT_SID_T_SOIL_3)\n\n#define CUR_SOIL_M_4_WDID        MAKE_WDID(WDAT_CV_DIRECT_DATA, WDAT_DU_SOIL_MOISTURE, WDAT_DT_CURRENT,   WDAT_ST_SOIL,   WDAT_SID_T_SOIL_4)\n#define DAY_HI_SOIL_M_4_WDID     MAKE_WDID(WDAT_CV_DIRECT_DATA, WDAT_DU_SOIL_MOISTURE, WDAT_DT_DAY_HIGH,  WDAT_ST_SOIL,   WDAT_SID_T_SOIL_4)\n#define DAY_LOW_SOIL_M_4_WDID    MAKE_WDID(WDAT_CV_DIRECT_DATA, WDAT_DU_SOIL_MOISTURE, WDAT_DT_DAY_LOW,   WDAT_ST_SOIL,   WDAT_SID_T_SOIL_4)\n#define MONTH_HI_SOIL_M_4_WDID   MAKE_WDID(WDAT_CV_DIRECT_DATA, WDAT_DU_SOIL_MOISTURE, WDAT_DT_MONTH_HIGH,WDAT_ST_SOIL,   WDAT_SID_T_SOIL_4)\n#define MONTH_LOW_SOIL_M_4_WDID  MAKE_WDID(WDAT_CV_DIRECT_DATA, WDAT_DU_SOIL_MOISTURE, WDAT_DT_MONTH_LOW, WDAT_ST_SOIL,   WDAT_SID_T_SOIL_4)\n#define YEAR_HI_SOIL_M_4_WDID    MAKE_WDID(WDAT_CV_DIRECT_DATA, WDAT_DU_SOIL_MOISTURE, WDAT_DT_YEAR_HIGH, WDAT_ST_SOIL,   WDAT_SID_T_SOIL_4)\n#define YEAR_LOW_SOIL_M_4_WDID   MAKE_WDID(WDAT_CV_DIRECT_DATA, WDAT_DU_SOIL_MOISTURE, WDAT_DT_YEAR_LOW,  WDAT_ST_SOIL,   WDAT_SID_T_SOIL_4)\n\n// Soil Temperature\n#define CUR_SOIL_T_1_WDID        MAKE_WDID(WDAT_CV_DIRECT_DATA, WDAT_DU_TEMP_DEG, WDAT_DT_CURRENT,   WDAT_ST_TEMPERATURE, WDAT_SID_T_SOIL_1)\n#define DAY_HI_SOIL_T_1_WDID     MAKE_WDID(WDAT_CV_DIRECT_DATA, WDAT_DU_TEMP_DEG, WDAT_DT_DAY_HIGH,  WDAT_ST_TEMPERATURE, WDAT_SID_T_SOIL_1)\n#define DAY_LOW_SOIL_T_1_WDID    MAKE_WDID(WDAT_CV_DIRECT_DATA, WDAT_DU_TEMP_DEG, WDAT_DT_DAY_LOW,   WDAT_ST_TEMPERATURE, WDAT_SID_T_SOIL_1)\n#define MONTH_HI_SOIL_T_1_WDID   MAKE_WDID(WDAT_CV_DIRECT_DATA, WDAT_DU_TEMP_DEG, WDAT_DT_MONTH_HIGH,WDAT_ST_TEMPERATURE, WDAT_SID_T_SOIL_1)\n#define MONTH_LOW_SOIL_T_1_WDID  MAKE_WDID(WDAT_CV_DIRECT_DATA, WDAT_DU_TEMP_DEG, WDAT_DT_MONTH_LOW, WDAT_ST_TEMPERATURE, WDAT_SID_T_SOIL_1)\n#define YEAR_HI_SOIL_T_1_WDID    MAKE_WDID(WDAT_CV_DIRECT_DATA, WDAT_DU_TEMP_DEG, WDAT_DT_YEAR_HIGH, WDAT_ST_TEMPERATURE, WDAT_SID_T_SOIL_1)\n#define YEAR_LOW_SOIL_T_1_WDID   MAKE_WDID(WDAT_CV_DIRECT_DATA, WDAT_DU_TEMP_DEG, WDAT_DT_YEAR_LOW,  WDAT_ST_TEMPERATURE, WDAT_SID_T_SOIL_1)\n\n#define CUR_SOIL_T_2_WDID        MAKE_WDID(WDAT_CV_DIRECT_DATA, WDAT_DU_TEMP_DEG, WDAT_DT_CURRENT,   WDAT_ST_TEMPERATURE, WDAT_SID_T_SOIL_2)\n#define DAY_HI_SOIL_T_2_WDID     MAKE_WDID(WDAT_CV_DIRECT_DATA, WDAT_DU_TEMP_DEG, WDAT_DT_DAY_HIGH,  WDAT_ST_TEMPERATURE, WDAT_SID_T_SOIL_2)\n#define DAY_LOW_SOIL_T_2_WDID    MAKE_WDID(WDAT_CV_DIRECT_DATA, WDAT_DU_TEMP_DEG, WDAT_DT_DAY_LOW,   WDAT_ST_TEMPERATURE, WDAT_SID_T_SOIL_2)\n#define MONTH_HI_SOIL_T_2_WDID   MAKE_WDID(WDAT_CV_DIRECT_DATA, WDAT_DU_TEMP_DEG, WDAT_DT_MONTH_HIGH,WDAT_ST_TEMPERATURE, WDAT_SID_T_SOIL_2)\n#define MONTH_LOW_SOIL_T_2_WDID  MAKE_WDID(WDAT_CV_DIRECT_DATA, WDAT_DU_TEMP_DEG, WDAT_DT_MONTH_LOW, WDAT_ST_TEMPERATURE, WDAT_SID_T_SOIL_2)\n#define YEAR_HI_SOIL_T_2_WDID    MAKE_WDID(WDAT_CV_DIRECT_DATA, WDAT_DU_TEMP_DEG, WDAT_DT_YEAR_HIGH, WDAT_ST_TEMPERATURE, WDAT_SID_T_SOIL_2)\n#define YEAR_LOW_SOIL_T_2_WDID   MAKE_WDID(WDAT_CV_DIRECT_DATA, WDAT_DU_TEMP_DEG, WDAT_DT_YEAR_LOW,  WDAT_ST_TEMPERATURE, WDAT_SID_T_SOIL_2)\n\n#define CUR_SOIL_T_3_WDID        MAKE_WDID(WDAT_CV_DIRECT_DATA, WDAT_DU_TEMP_DEG, WDAT_DT_CURRENT,   WDAT_ST_TEMPERATURE, WDAT_SID_T_SOIL_3)\n#define DAY_HI_SOIL_T_3_WDID     MAKE_WDID(WDAT_CV_DIRECT_DATA, WDAT_DU_TEMP_DEG, WDAT_DT_DAY_HIGH,  WDAT_ST_TEMPERATURE, WDAT_SID_T_SOIL_3)\n#define DAY_LOW_SOIL_T_3_WDID    MAKE_WDID(WDAT_CV_DIRECT_DATA, WDAT_DU_TEMP_DEG, WDAT_DT_DAY_LOW,   WDAT_ST_TEMPERATURE, WDAT_SID_T_SOIL_3)\n#define MONTH_HI_SOIL_T_3_WDID   MAKE_WDID(WDAT_CV_DIRECT_DATA, WDAT_DU_TEMP_DEG, WDAT_DT_MONTH_HIGH,WDAT_ST_TEMPERATURE, WDAT_SID_T_SOIL_3)\n#define MONTH_LOW_SOIL_T_3_WDID  MAKE_WDID(WDAT_CV_DIRECT_DATA, WDAT_DU_TEMP_DEG, WDAT_DT_MONTH_LOW, WDAT_ST_TEMPERATURE, WDAT_SID_T_SOIL_3)\n#define YEAR_HI_SOIL_T_3_WDID    MAKE_WDID(WDAT_CV_DIRECT_DATA, WDAT_DU_TEMP_DEG, WDAT_DT_YEAR_HIGH, WDAT_ST_TEMPERATURE, WDAT_SID_T_SOIL_3)\n#define YEAR_LOW_SOIL_T_3_WDID   MAKE_WDID(WDAT_CV_DIRECT_DATA, WDAT_DU_TEMP_DEG, WDAT_DT_YEAR_LOW,  WDAT_ST_TEMPERATURE, WDAT_SID_T_SOIL_3)\n\n#define CUR_SOIL_T_4_WDID        MAKE_WDID(WDAT_CV_DIRECT_DATA, WDAT_DU_TEMP_DEG, WDAT_DT_CURRENT,   WDAT_ST_TEMPERATURE, WDAT_SID_T_SOIL_4)\n#define DAY_HI_SOIL_T_4_WDID     MAKE_WDID(WDAT_CV_DIRECT_DATA, WDAT_DU_TEMP_DEG, WDAT_DT_DAY_HIGH,  WDAT_ST_TEMPERATURE, WDAT_SID_T_SOIL_4)\n#define DAY_LOW_SOIL_T_4_WDID    MAKE_WDID(WDAT_CV_DIRECT_DATA, WDAT_DU_TEMP_DEG, WDAT_DT_DAY_LOW,   WDAT_ST_TEMPERATURE, WDAT_SID_T_SOIL_4)\n#define MONTH_HI_SOIL_T_4_WDID   MAKE_WDID(WDAT_CV_DIRECT_DATA, WDAT_DU_TEMP_DEG, WDAT_DT_MONTH_HIGH,WDAT_ST_TEMPERATURE, WDAT_SID_T_SOIL_4)\n#define MONTH_LOW_SOIL_T_4_WDID  MAKE_WDID(WDAT_CV_DIRECT_DATA, WDAT_DU_TEMP_DEG, WDAT_DT_MONTH_LOW, WDAT_ST_TEMPERATURE, WDAT_SID_T_SOIL_4)\n#define YEAR_HI_SOIL_T_4_WDID    MAKE_WDID(WDAT_CV_DIRECT_DATA, WDAT_DU_TEMP_DEG, WDAT_DT_YEAR_HIGH, WDAT_ST_TEMPERATURE, WDAT_SID_T_SOIL_4)\n#define YEAR_LOW_SOIL_T_4_WDID   MAKE_WDID(WDAT_CV_DIRECT_DATA, WDAT_DU_TEMP_DEG, WDAT_DT_YEAR_LOW,  WDAT_ST_TEMPERATURE, WDAT_SID_T_SOIL_4)\n\n// Leaf Wetness\n#define CUR_LEAF_W_1_WDID        MAKE_WDID(WDAT_CV_DIRECT_DATA, WDAT_DU_LEAF_WET, WDAT_DT_CURRENT,   WDAT_ST_LEAF,        WDAT_SID_T_LEAF_1)\n#define DAY_HI_LEAF_W_1_WDID     MAKE_WDID(WDAT_CV_DIRECT_DATA, WDAT_DU_LEAF_WET, WDAT_DT_DAY_HIGH,  WDAT_ST_LEAF,        WDAT_SID_T_LEAF_1)\n#define DAY_LOW_LEAF_W_1_WDID    MAKE_WDID(WDAT_CV_DIRECT_DATA, WDAT_DU_LEAF_WET, WDAT_DT_DAY_LOW,   WDAT_ST_LEAF,        WDAT_SID_T_LEAF_1)\n#define MONTH_HI_LEAF_W_1_WDID   MAKE_WDID(WDAT_CV_DIRECT_DATA, WDAT_DU_LEAF_WET, WDAT_DT_MONTH_HIGH,WDAT_ST_LEAF,        WDAT_SID_T_LEAF_1)\n#define MONTH_LOW_LEAF_W_1_WDID  MAKE_WDID(WDAT_CV_DIRECT_DATA, WDAT_DU_LEAF_WET, WDAT_DT_MONTH_LOW, WDAT_ST_LEAF,        WDAT_SID_T_LEAF_1)\n#define YEAR_HI_LEAF_W_1_WDID    MAKE_WDID(WDAT_CV_DIRECT_DATA, WDAT_DU_LEAF_WET, WDAT_DT_YEAR_HIGH, WDAT_ST_LEAF,        WDAT_SID_T_LEAF_1)\n#define YEAR_LOW_LEAF_W_1_WDID   MAKE_WDID(WDAT_CV_DIRECT_DATA, WDAT_DU_LEAF_WET, WDAT_DT_YEAR_LOW,  WDAT_ST_LEAF,        WDAT_SID_T_LEAF_1)\n\n#define CUR_LEAF_W_2_WDID        MAKE_WDID(WDAT_CV_DIRECT_DATA, WDAT_DU_LEAF_WET, WDAT_DT_CURRENT,   WDAT_ST_LEAF,        WDAT_SID_T_LEAF_2)\n#define DAY_HI_LEAF_W_2_WDID     MAKE_WDID(WDAT_CV_DIRECT_DATA, WDAT_DU_LEAF_WET, WDAT_DT_DAY_HIGH,  WDAT_ST_LEAF,        WDAT_SID_T_LEAF_2)\n#define DAY_LOW_LEAF_W_2_WDID    MAKE_WDID(WDAT_CV_DIRECT_DATA, WDAT_DU_LEAF_WET, WDAT_DT_DAY_LOW,   WDAT_ST_LEAF,        WDAT_SID_T_LEAF_2)\n#define MONTH_HI_LEAF_W_2_WDID   MAKE_WDID(WDAT_CV_DIRECT_DATA, WDAT_DU_LEAF_WET, WDAT_DT_MONTH_HIGH,WDAT_ST_LEAF,        WDAT_SID_T_LEAF_2)\n#define MONTH_LOW_LEAF_W_2_WDID  MAKE_WDID(WDAT_CV_DIRECT_DATA, WDAT_DU_LEAF_WET, WDAT_DT_MONTH_LOW, WDAT_ST_LEAF,        WDAT_SID_T_LEAF_2)\n#define YEAR_HI_LEAF_W_2_WDID    MAKE_WDID(WDAT_CV_DIRECT_DATA, WDAT_DU_LEAF_WET, WDAT_DT_YEAR_HIGH, WDAT_ST_LEAF,        WDAT_SID_T_LEAF_2)\n#define YEAR_LOW_LEAF_W_2_WDID   MAKE_WDID(WDAT_CV_DIRECT_DATA, WDAT_DU_LEAF_WET, WDAT_DT_YEAR_LOW,  WDAT_ST_LEAF,        WDAT_SID_T_LEAF_2)\n\n// Leaf Temperature\n#define CUR_LEAF_T_1_WDID        MAKE_WDID(WDAT_CV_DIRECT_DATA, WDAT_DU_TEMP_DEG, WDAT_DT_CURRENT,   WDAT_ST_TEMPERATURE, WDAT_SID_T_LEAF_1)\n#define DAY_HI_LEAF_T_1_WDID     MAKE_WDID(WDAT_CV_DIRECT_DATA, WDAT_DU_TEMP_DEG, WDAT_DT_DAY_HIGH,  WDAT_ST_TEMPERATURE, WDAT_SID_T_LEAF_1)\n#define DAY_LOW_LEAF_T_1_WDID    MAKE_WDID(WDAT_CV_DIRECT_DATA, WDAT_DU_TEMP_DEG, WDAT_DT_DAY_LOW,   WDAT_ST_TEMPERATURE, WDAT_SID_T_LEAF_1)\n#define MONTH_HI_LEAF_T_1_WDID   MAKE_WDID(WDAT_CV_DIRECT_DATA, WDAT_DU_TEMP_DEG, WDAT_DT_MONTH_HIGH,WDAT_ST_TEMPERATURE, WDAT_SID_T_LEAF_1)\n#define MONTH_LOW_LEAF_T_1_WDID  MAKE_WDID(WDAT_CV_DIRECT_DATA, WDAT_DU_TEMP_DEG, WDAT_DT_MONTH_LOW, WDAT_ST_TEMPERATURE, WDAT_SID_T_LEAF_1)\n#define YEAR_HI_LEAF_T_1_WDID    MAKE_WDID(WDAT_CV_DIRECT_DATA, WDAT_DU_TEMP_DEG, WDAT_DT_YEAR_HIGH, WDAT_ST_TEMPERATURE, WDAT_SID_T_LEAF_1)\n#define YEAR_LOW_LEAF_T_1_WDID   MAKE_WDID(WDAT_CV_DIRECT_DATA, WDAT_DU_TEMP_DEG, WDAT_DT_YEAR_LOW,  WDAT_ST_TEMPERATURE, WDAT_SID_T_LEAF_1)\n\n#define CUR_LEAF_T_2_WDID        MAKE_WDID(WDAT_CV_DIRECT_DATA, WDAT_DU_TEMP_DEG, WDAT_DT_CURRENT,   WDAT_ST_TEMPERATURE, WDAT_SID_T_LEAF_2)\n#define DAY_HI_LEAF_T_2_WDID     MAKE_WDID(WDAT_CV_DIRECT_DATA, WDAT_DU_TEMP_DEG, WDAT_DT_DAY_HIGH,  WDAT_ST_TEMPERATURE, WDAT_SID_T_LEAF_2)\n#define DAY_LOW_LEAF_T_2_WDID    MAKE_WDID(WDAT_CV_DIRECT_DATA, WDAT_DU_TEMP_DEG, WDAT_DT_DAY_LOW,   WDAT_ST_TEMPERATURE, WDAT_SID_T_LEAF_2)\n#define MONTH_HI_LEAF_T_2_WDID   MAKE_WDID(WDAT_CV_DIRECT_DATA, WDAT_DU_TEMP_DEG, WDAT_DT_MONTH_HIGH,WDAT_ST_TEMPERATURE, WDAT_SID_T_LEAF_2)\n#define MONTH_LOW_LEAF_T_2_WDID  MAKE_WDID(WDAT_CV_DIRECT_DATA, WDAT_DU_TEMP_DEG, WDAT_DT_MONTH_LOW, WDAT_ST_TEMPERATURE, WDAT_SID_T_LEAF_2)\n#define YEAR_HI_LEAF_T_2_WDID    MAKE_WDID(WDAT_CV_DIRECT_DATA, WDAT_DU_TEMP_DEG, WDAT_DT_YEAR_HIGH, WDAT_ST_TEMPERATURE, WDAT_SID_T_LEAF_2)\n#define YEAR_LOW_LEAF_T_2_WDID   MAKE_WDID(WDAT_CV_DIRECT_DATA, WDAT_DU_TEMP_DEG, WDAT_DT_YEAR_LOW,  WDAT_ST_TEMPERATURE, WDAT_SID_T_LEAF_2)\n\n// Other values\n#define CONSOLE_BATT_WDID        MAKE_WDID(WDAT_CV_DIRECT_DATA, WDAT_DU_SCALAR,   WDAT_DT_CURRENT,   WDAT_ST_NUMBER,      WDAT_SID_CON_BATT)\n#define TX_BATT_WDID             MAKE_WDID(WDAT_CV_DIRECT_DATA, WDAT_DU_SCALAR,   WDAT_DT_CURRENT,   WDAT_ST_NUMBER,      WDAT_SID_TX_BATT)\n#define REPEATER_BATT_WDID       MAKE_WDID(WDAT_CV_DIRECT_DATA, WDAT_DU_SCALAR,   WDAT_DT_CURRENT,   WDAT_ST_NUMBER,      WDAT_SID_REP_BATT)\n#define FORECAST_WDID            MAKE_WDID(WDAT_CV_DIRECT_DATA, WDAT_DU_SCALAR,   WDAT_DT_CURRENT,   WDAT_ST_NUMBER,      WDAT_SID_FORECAST_CODE)\n#define FORECAST_ICON_WDID       MAKE_WDID(WDAT_CV_DIRECT_DATA, WDAT_DU_SCALAR,   WDAT_DT_CURRENT,   WDAT_ST_NUMBER,      WDAT_SID_FORECAST_ICON)\n#define SUNRISE_WDID             MAKE_WDID(WDAT_CV_DIRECT_DATA, WDAT_DU_TIME,     WDAT_DT_CURRENT,   WDAT_ST_TIME,        WDAT_SID_SUNRISE)\n#define SUNSET_WDID              MAKE_WDID(WDAT_CV_DIRECT_DATA, WDAT_DU_TIME,     WDAT_DT_CURRENT,   WDAT_ST_TIME,        WDAT_SID_SUNSET)\n\n// LOOP2 data\n#define WIND_2MIN_AVG_WDID         MAKE_WDID(WDAT_CV_DIRECT_DATA, WDAT_DU_SPEED,    WDAT_DT_CURRENT,    WDAT_ST_SPEED,       WDAT_DT_2MIN_AVG)    \n#define WIND_GUST_10MIN_WDID       MAKE_WDID(WDAT_CV_DIRECT_DATA, WDAT_DU_SPEED,    WDAT_DT_CURRENT,   WDAT_ST_SPEED,     WDAT_DT_10MIN_HIGH)    \n#define LAST_HOUR_RAIN_WDID      MAKE_WDID(WDAT_CV_DIRECT_DATA, WDAT_DU_WATER_ACCUM, WDAT_DT_1HR_ACCUM,   WDAT_ST_RAIN,        WDAT_SID_DEFAULT_SENSOR)    \n#define LAST_24HOUR_RAIN_WDID    MAKE_WDID(WDAT_CV_DIRECT_DATA, WDAT_DU_WATER_ACCUM, WDAT_DT_24HR_ACCUM,  WDAT_ST_RAIN,        WDAT_SID_DEFAULT_SENSOR)    \n#define BAR_ALTIMETER_WDID       MAKE_WDID(WDAT_CV_DIRECT_DATA, WDAT_DU_PRESSURE,    WDAT_DT_CURRENT,  WDAT_ST_BAROMETER,   WDAT_SID_BAR_ALTIMETER)"
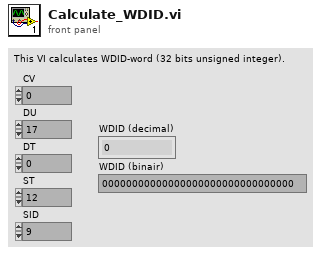
[diagram p1: front panel]
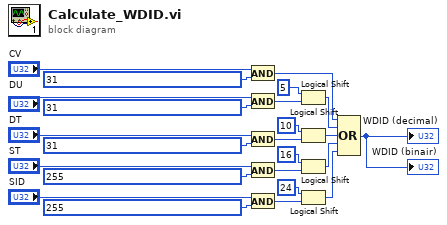
[diagram p0: block diagram]
diagram:
  n1 = And(x="CV", y=u32 31) -> (x .and. y?=w14:u32)
  n2 = And(x="DU", y=u32 31) -> (x .and. y?=w8:u32)
  n3 = And(x="DT", y=u32 31) -> (x .and. y?=w4:u32)
  n4 = And(x="ST", y=u32 255) -> (x .and. y?=w6:u32)
  n5 = And(x="SID", y=u32 255) -> (x .and. y?=w2:u32)
  n6 = Logical Shift(y=u32 5 ("x"), x=w8) -> (x << y=w13:u32)
  n7 = Logical Shift(y=u32 10 ("x"), x=w4) -> (x << y=w12:u32)
  n8 = Logical Shift(y=u32 16 ("x"), x=w6) -> (x << y=w10:u32)
  n9 = Logical Shift(y=u32 24 ("x"), x=w2) -> (x << y=w9:u32)
  n10 = Compound Arithmetic op=OR(w14, w13, w12, w10, w9) -> (→"WDID (decimal)" →"WDID (binair)":u32)
